vi "DopplerSVD_3D.vi"(0 "Choose Directory":path) -> ()   [LabVIEW 2022 SP3]
uses:
  <vilib>/Analysis/NI_AALPro.lvlib
  <vilib>/Analysis/Matrix/NI_Matrix.lvlib
  <vilib>/Analysis/Matrix/Numeric/Conversions/Matrix To Array - CM.vi
  <vilib>/Analysis/2dsp.llb/Complex FFT.vi
panel:
  in  "ms between frames":u32=100
  in  "Calc Spec Peaks":bool
  in  "animate":bool
  out "Peak V":sgl[][](graph)
  in  "read?":bool
  out "Waveform Graph":dbl[](graph)
  out "Complex output array":csg[][][](array[numeric])
  in  "image to display":i32
  in  "SV cut off":i32
  in  "stop":bool
  out "Raw data":dbl[][](graph)
  in  "Window Increment":i32=64
  in  "Window length":i32=64
  out "Doppler Signal":dbl[][](graph)
  in  "Parse":u16=1
  in  "Filter Prams":T1={"low cutoff"=5, "order"=81, "high cutoff"=35}
  in  "Type of Mean":u16(ring)=3 items=["Mean from lines", "Mean just lines", "Poly Mean", "No mean", "Filter"]
  in  "file ext":string="*IQSum_B3*"
  out "Numeric":i32
  in  "Use Selected Files":bool
  in  "Listbox":i32[](listbox)
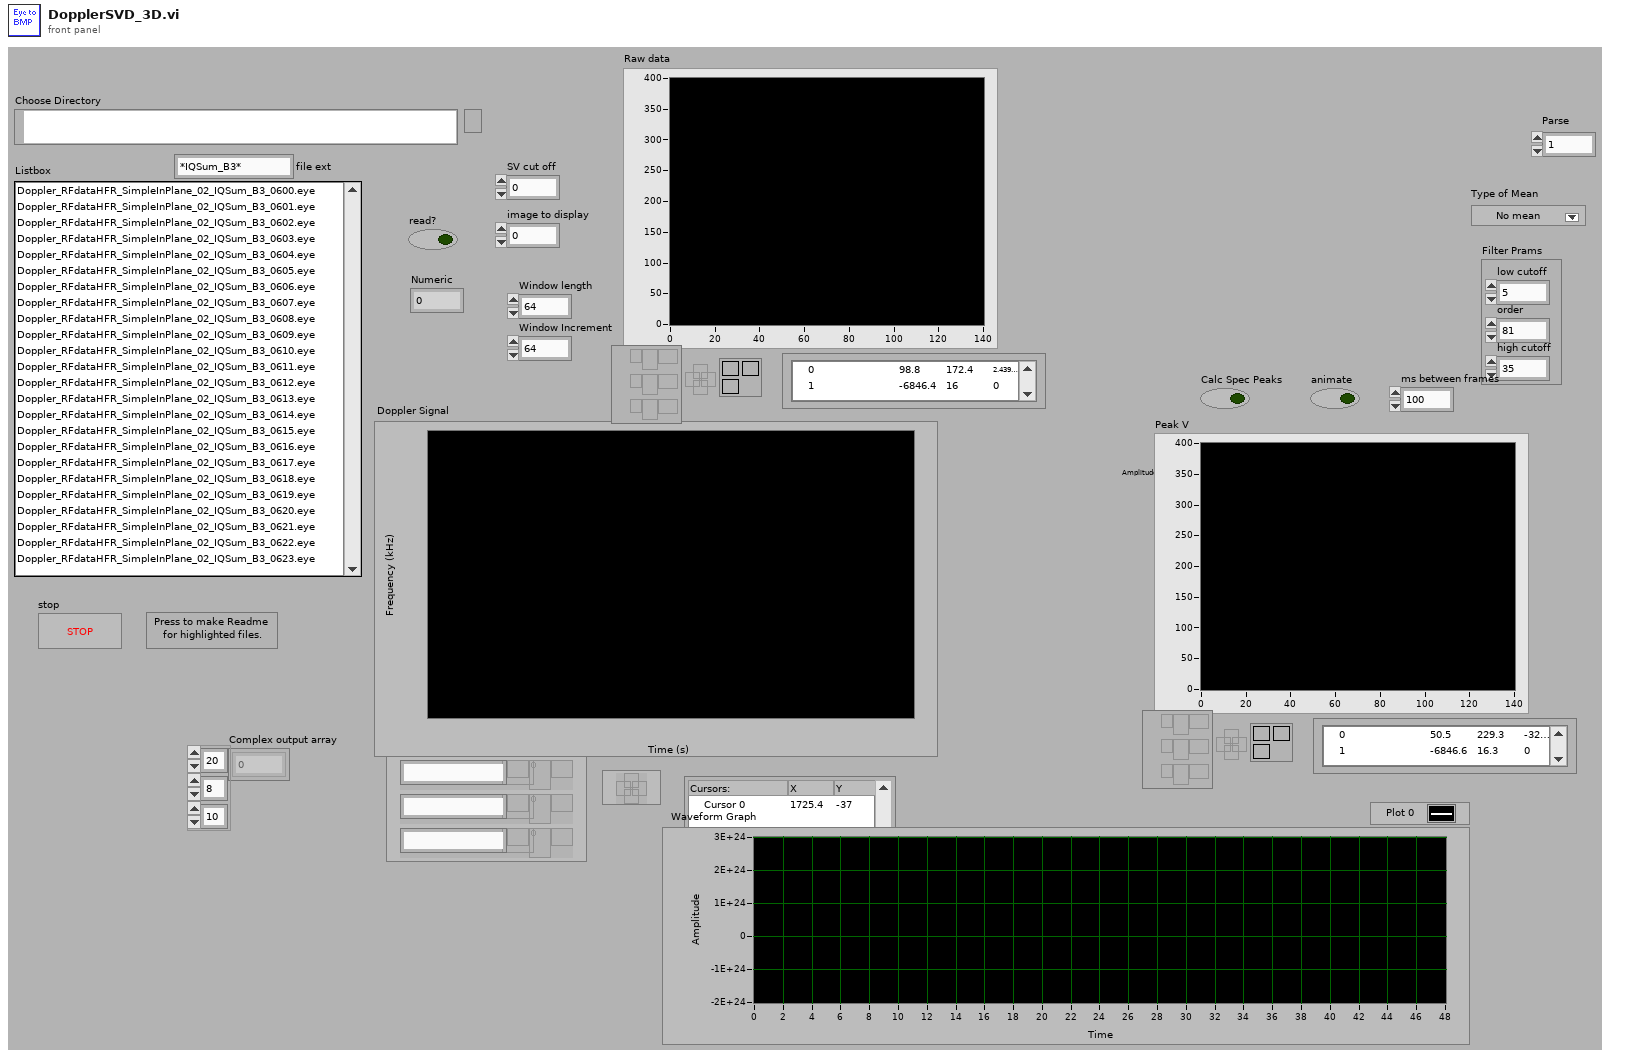
[diagram p1: front panel]
types:
  T1 = cluster{"low cutoff":i32, "order":i32, "high cutoff":i32}
  T2 = typedef "Header.ctl" = cluster{"header info":cluster{"Header":string, "Head length":i16}, "A/D info":cluster{"# rf points per line":u16, "# lines per scan":u16, "sample rate MHz":u16, "# A/D bits":i16, "# bytes per A/D":u16, "TGC Flag":u16, "A/D Type":string}, "Tranducer Info":cluster{"bandwidth":sgl, "center freq":sgl, "start freq":sgl, "ID":i32}, "Scan Info":cluster{"delay":sgl, "pivot distance":sgl, "sector scan angle":sgl, "operator":string, "Scan Mode":string, "location":string}, "Time/Date Info":cluster{"date":string, "time":string}, "RF Info":cluster{"RF file name":string, "RF file att":string, "RF cal file name":string, "RF cal file att":string}, "Patient Info":cluster{"ID":string, "extended ID":string, "age":u16, "sex":string, "previously\nscanned":string, "PSA":sgl, "LOS":u8, "Ethnicty 2":u8, "Race":u8}, "Tissue Type":cluster{"organ":i16, "disease type":i16, "disease location":i16, "IQ_pts":u16, "RcvBuffer":u8, "RcvFrame":u16, "IQBuff":u8, "IQFrame":u16, "IQPage":u8}, "Votage scaling":cluster{"Digitizer (dB)":sgl, "Gain (dB)":sgl, "Atten (dB)":sgl}, "Comment":string, "Misc Info":cluster{"avg num":u16, "c speed":i16, "Div By or SF zones":i16, "XMIT CHS":u8, "RCV CHS":u8, "Xmit angle":sgl}, "Therapy Parameters":cluster{"Theraputic Freq (MHz)":sgl, "Time on (s)":sgl, "Therapy amplitude (mV)":sgl, "Lines Before":u16, "Lines After":u16}, "Scan Settings":cluster{"Energy (uJ or V)":u8, "Damp (Ohm) or Fc":u8, "HP Filt (KHz)":u8, "LP Filt (MHz)":u8, "Gain (db)":u8, "prf (kHz)":sgl, "Distance between\nscan lines (um)":u16, "Distance between\nscan planes (um)":u16, "Scan line gap (um)":sgl, "Scan plane gap (um)":sgl}, "Compression Parameters":cluster{"F1 (MHz)":sgl, "F2 (MHz)":sgl, "% taper":sgl, "duration":sgl}, "Patient Info Xtra":cluster{"First Name":string, "Last Name":string, "Notes":string}, "ROI Box":u16[]}
  T3 = cluster{cluster{dbl, u16}, dbl, dbl, "delay":sgl, "delay":sgl, dbl, dbl}
  T4 = typedef "NI_Matrix.lvlib/ComplexMatrix.ctl" = cdb[][]
  T5 = cluster{"Vector S":cdb[], "Matrix V":T4, "Spectra":dbl[][], "indexes":i32[]}
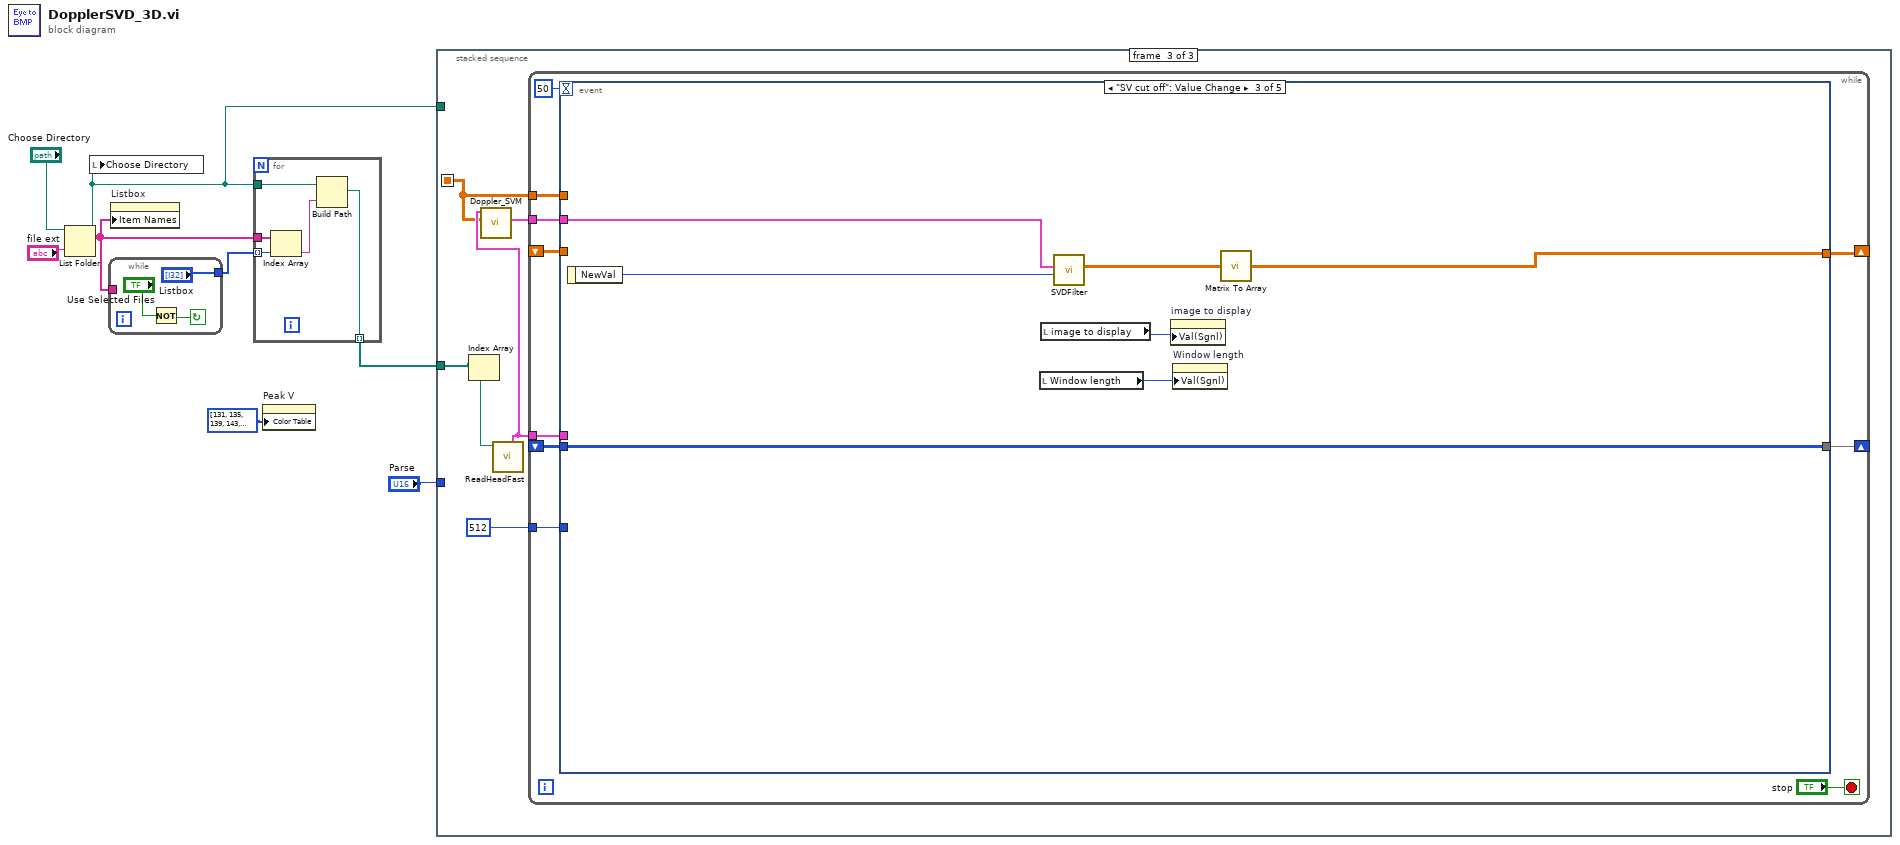
[diagram p0: block diagram]
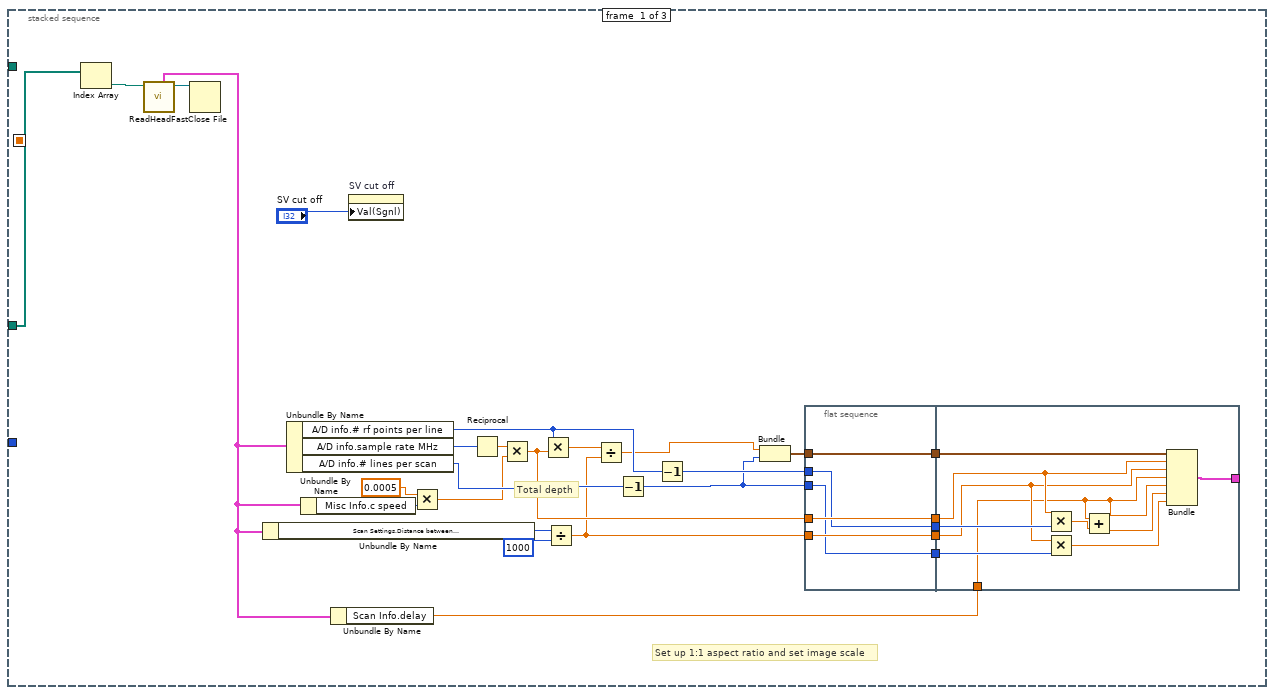
[diagram p2: hidden frame]
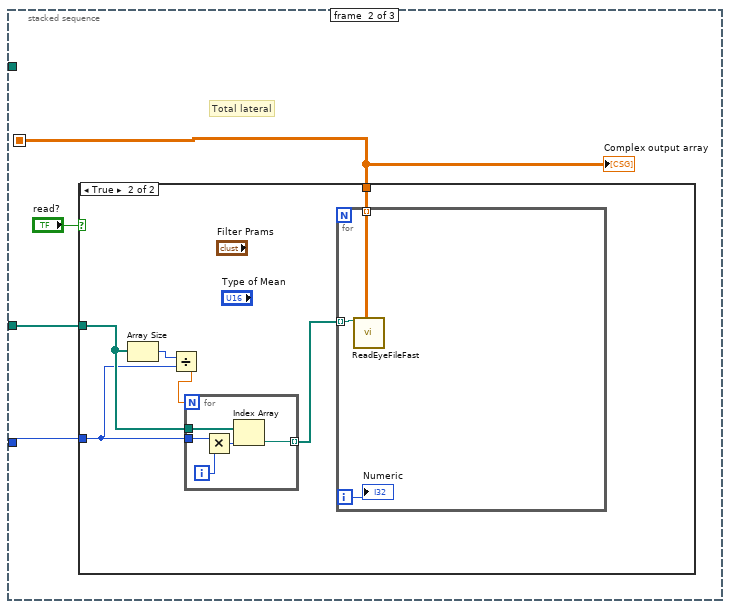
[diagram p3: hidden frame]
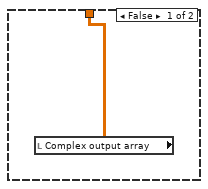
[diagram p4: hidden frame]
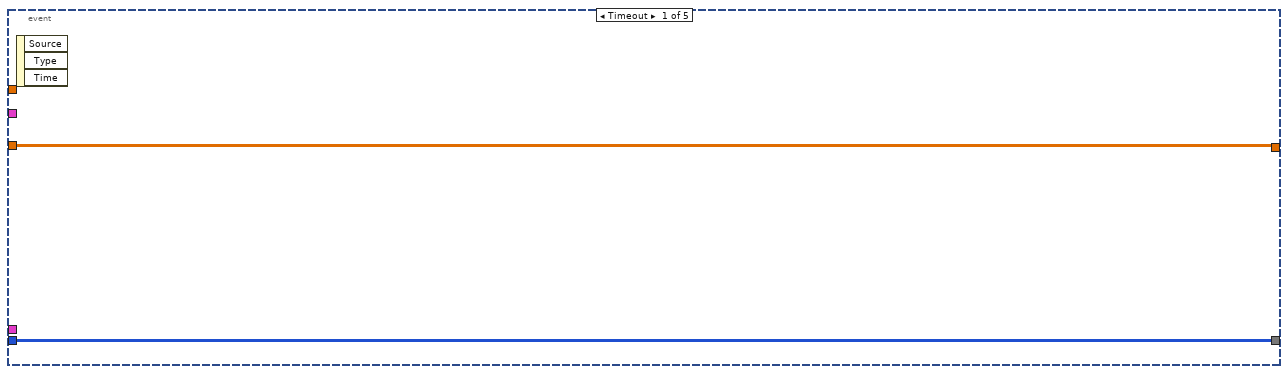
[diagram p5: hidden frame]
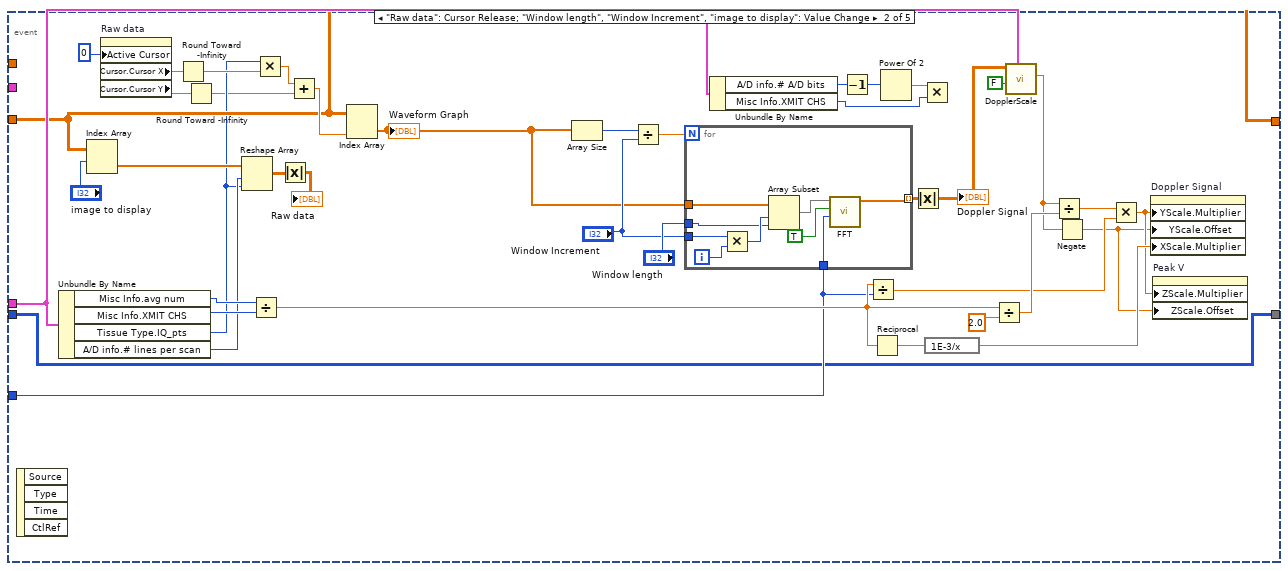
[diagram p6: hidden frame]
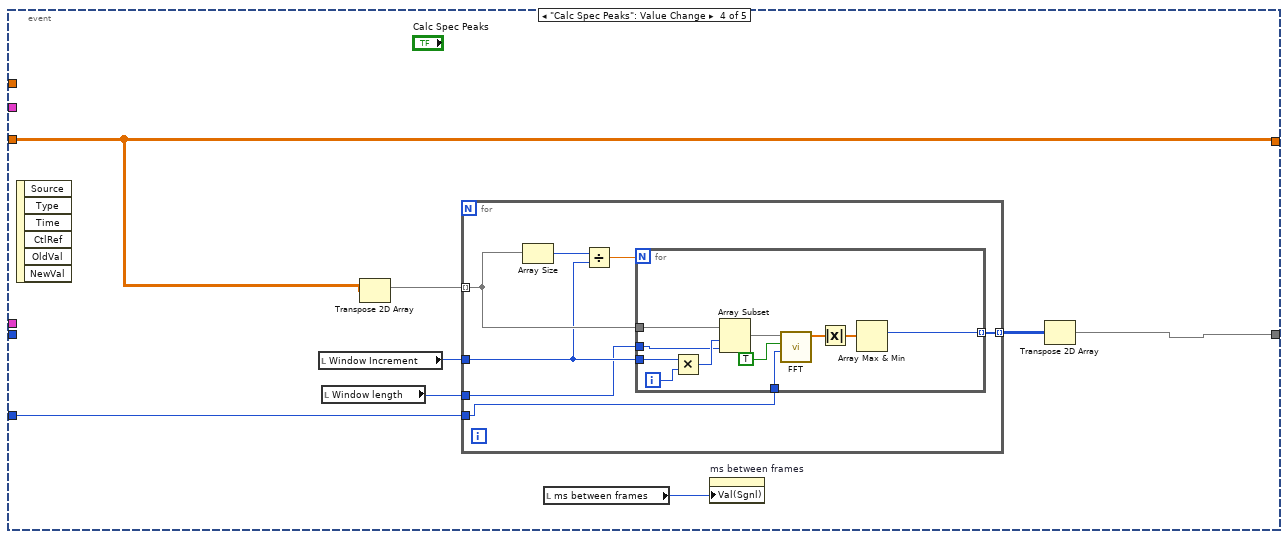
[diagram p7: hidden frame]
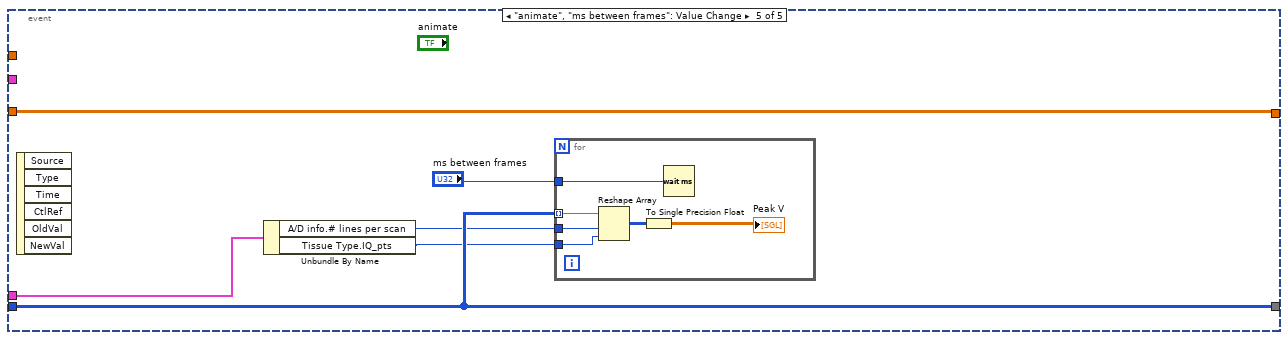
[diagram p8: hidden frame]
diagram:
  n1 = List Folder(path="Choose Directory", pattern="file ext") -> (path out=w5:path, filenames=w8:string[])  [unwired: 1 in, 3 out]
  n2 = local write "Choose Directory"(w5) -> ()
  n3 = while {
    tunnel: ["Listbox"] -> w7
    tunnel: w8 -> [_]
    stop <- w11 continue-if-true
    n4 = Not(x="Use Selected Files") -> (.not. x?=w11:bool)
  }
  n5 = property on="Listbox" class="LstBox (strict)"("Item Names"=w8) -> ()  [unwired: 2 in, 2 out]
  n6 = for {
    tunnel: w8 -> [w16]
    tunnel: w7 -> [w15] mode=indexing
    tunnel: [w12] -> w2 mode=indexing
    tunnel: w5 -> [w13]
    n7 = Index Array(array=w16, index=w15) -> (element=w14:string)
    n8 = Build Path(base path=w13, name or relative path=w14) -> (appended path=w12:path)
  }
  n9 = property on="Peak V" class="IntGraph (strict)"("Color Table"=u32[] [131, 135, 139, 143, 147, 151, 155, 159, 163, 167, 171, 175, 179, 183, 187, 191, 195, 199, 203, 207, 211, 215, 219, 223, 227, 231, 235, 239, 243, 247, 251, 255, 1279, 2303, 3327, 4351, 5375, 6399, 7423, 8447, 9471, 10495, 11519, 12543, 13567, 14591, 15615, 16639, 17663, 18687, 19711, 20735, 21759, 22783, 23807, 24831, 25855, 26879, 27903, 28927, 29951, 30975, 31999, 33023, 33791, 34815, 35839, 36863, 37887, 38911, 39935, 40959, 41983, 43007, 44031, 45055, 46079, 47103, 48127, 49151, 50175, 51199, 52223, 53247, 54271, 55295, 56319, 57343, 58367, 59391, 60415, 61439, 62463, 63487, 64511, 65535, 327675, 589815, 851955, 1114095, 1376235, 1638375, 1900515, 2162655, 2424795, 2686935, 2949075, 3211215, 3473355, 3735495, 3997635, 4259775, 4521915, 4784055, 5046195, 5308335, 5570475, 5832615, 6094755, 6356895, 6619035, 6881175, 7143315, 7405455, 7667595, 7929735, 8191875, 8454016, 8650620, 8912760, 9174900, 9437040, 9699180, 9961320, 10223460, 10485600, 10747740, 11009880, 11272020, 11534160, 11796300, 12058440, 12320580, 12582720, 12844860, 13107000, 13369140, 13631280, 13893420, 14155560, 14417700, 14679840, 14941980, 15204120, 15466260, 15728400, 15990540, 16252680, 16514820, 16776960, 16775936, 16774912, 16773888, 16772864, 16771840, 16770816, 16769792, 16768768, 16767744, 16766720, 16765696, 16764672, 16763648, 16762624, 16761600, 16760576, 16759552, 16758528, 16757504, 16756480, 16755456, 16754432, 16753408, 16752384, 16751360, 16750336, 16749312, 16748288, 16747264, 16746240, 16745216, 16744448, 16743424, 16742400, 16741376, 16740352, 16739328, 16738304, 16737280, 16736256, 16735232, 16734208, 16733184, 16732160, 16731136, 16730112, 16729088, 16728064, 16727040, 16726016, 16724992, 16723968, 16722944, 16721920, 16720896, 16719872, 16718848, 16717824, 16716800, 16715776, 16714752, 16713728, 16712704, 16711680, 16449536, 16187392, 15925248, 15663104, 15400960, 15138816, 14876672, 14614528, 14352384, 14090240, 13828096, 13565952, 13303808, 13041664, 12779520, 12517376, 12255232, 11993088, 11730944, 11468800, 11206656, 10944512, 10682368, 10420224, 10158080, 9895936, 9633792, 9371648, 9109504, 8847360, 8585216, 8388608] ("Array")) -> ()  [unwired: 2 in, 2 out]
  n10 = stacked-sequence {
    seq-local: [_ w60 _] -> [_ _ w79]
    tunnel: w2 -> [w41 w62 w82]
    tunnel: w5 -> [_ _ _]
    tunnel: "Parse" -> [_ w61 _]
    frame #0 {
      # "Set up 1:1 aspect ratio and set image scale"
      # "Total depth"
      n11 = Index Array(array=w41) -> (element=w43:path)  [unwired: 1 in]
      n12 = call "ReadHeadFast.vi"("new file path"=w43) -> ("refnum out"=w42:refnum<file>, "Header In"=w40:T2)  [unwired: 7 in, 2 out]
      n13 = Close File(refnum=w42) -> ()  [unwired: 1 in, 2 out]
      n14 = Unbundle By Name(w40) -> ("Scan Settings.Distance between\nscan lines (um)"=w27:u16)
      n15 = Unbundle By Name(w40) -> ("A/D info.# rf points per line"=w30:u16, "A/D info.sample rate MHz"=w32:u16, "A/D info.# lines per scan"=w29:u16)
      n16 = Unbundle By Name(w40) -> ("Misc Info.c speed"=w26:i16)
      n17 = Unbundle By Name(w40) -> ("Scan Info.delay"=w22:sgl)
      n18 = property on="SV cut off" class="DigNum (strict)"("Val(Sgnl)"="SV cut off") -> ()  [unwired: 2 in, 2 out]
      n19 = Multiply(x=0.0005, y=w26) -> (x*y=w24:dbl)
      n20 = Reciprocal(x=w32) -> (1/x=w33:dbl)
      n21 = Multiply(x=w33, y=w24) -> (x*y=w23:dbl)
      n22 = Multiply(x=w30, y=w23) -> (x*y=w31:dbl)
      n23 = Divide(x=w27, y=1000) -> (x/y=w21:dbl)
      n24 = Divide(x=w31, y=w21) -> (x/y=w19:dbl)
      n25 = Decrement(x=w29) -> (x-1=w18:u16)
      n26 = Decrement(x=w30) -> (x-1=w28:u16)
      n27 = Bundle(w19, w18) -> (w20:cluster{dbl, u16})  [unwired: 1 out]
      n28 = flat-sequence {
        tunnel: w28 -> [w45]
        tunnel: w18 -> [w46]
        tunnel: w20 -> [w44]
        tunnel: [w48] -> w39
        tunnel: w23 -> [w48]
        tunnel: [w47] -> w38
        tunnel: w21 -> [w47]
        tunnel: [w46] -> w37
        tunnel: [w45] -> w36
        tunnel: [w44] -> w35
        tunnel: w39 -> [w54]
        tunnel: w22 -> [w52]
        tunnel: w38 -> [w53]
        tunnel: w37 -> [w58]
        tunnel: w36 -> [w57]
        tunnel: w35 -> [w55]
        tunnel: [w49] -> _
        frame #0 {
        }
        frame #1 {
          n29 = Multiply(x=w54, y=w57) -> (x*y=w56:dbl)
          n30 = Multiply(x=w53, y=w58) -> (x*y=w50:dbl)
          n31 = Add(x=w52, y=w56) -> (x+y=w51:dbl)
          n32 = Bundle(w55, w54, w53, "delay"=w52, "delay"=w52, w51, w50) -> (w49:T3)  [unwired: 1 out]
        }
      }
    }
    frame #1 {
      # "Total lateral"
      n33 = case shown="True" "read?" {
        tunnel: w62 -> [_ w67]
        tunnel: w61 -> [_ w64]
        tunnel: [w63 w65] -> w60
        frame False {
          n34 = local read "Complex output array"() -> (w63:csg[][][])
        }
        frame True {
          n35 = Array Size(array=w67) -> (size(s)=w69:i32)
          n36 = Divide(x=w69, y=w64) -> (x/y=w68:dbl)
          n37 = for {
            N: w68 -> [_]
            tunnel: w67 -> [w73]
            tunnel: w64 -> [w72]
            tunnel: [w71] -> w66 mode=indexing
            i -> [w74]
            n38 = Multiply(x=w72, y=w74) -> (x*y=w70:i32)
            n39 = Index Array(array=w73, index=w70) -> (element=w71:path)
          }
          n40 = for {
            tunnel: w66 -> [w77] mode=indexing
            tunnel: [w75] -> w65 mode=indexing
            i -> [w76]
            n41 = call "ReadEyeFileFast.vi"("new file path"=w77) -> ("Complex output array"=w75:csg[][])  [unwired: 1 in, 17 out]
            "Numeric" <- w76
          }
        }
      }
      "Complex output array" <- w60
    }
    frame #2 {
      n42 = Index Array(array=w82) -> (element=w83:path)  [unwired: 1 in]
      n43 = call "ReadHeadFast.vi"("new file path"=w83) -> ("Header In"=w81:T2)  [unwired: 7 in, 3 out]
      n44 = call "Doppler_SVM.vi"("Input Array"=w79, "Header In"=w81) -> ("output cluster"=w80:T5)  [unwired: 8 in, 1 out]
      n45 = while {
        tunnel: w81 -> [w91]
        tunnel: w80 -> [w90]
        shift-right: [w89] -> _
        shift-left: _ -> [w88]
        tunnel: w79 -> [w87]
        shift-right: [w86] -> _
        shift-left: _ -> [w85]
        tunnel: 512 ("FFT size") -> [w84]
        stop <- "stop" stop-if-true
        n46 = event shown="[2] \"SV cut off\": Value Change" {
          selector: _ -> [_ _ _ _ _]
          dyn-events: _ -> [_ _ _ _ _]
          timeout: 50 -> [_ _ _ _ _]
          tunnel: w91 -> [_ w114 _ _ w182]
          tunnel: w90 -> [_ _ w152 _ _]
          tunnel: [w95 w108 w147 w160 w184] -> w89
          tunnel: w88 -> [w95 w108 _ w160 w184]
          tunnel: w87 -> [_ _ _ _ _]
          tunnel: [w94 w96 w146 w154 w183] -> w86
          tunnel: w85 -> [w94 w96 w146 _ w183]
          tunnel: w84 -> [_ w97 _ w155 _]
          event Timeout {
            n47 = event-data() -> ()  [unwired: 1 in, 3 out]
          }
          event "Raw data": Cursor Release; "Window length", "Window Increment", "image to display": Value Change {
            n48 = event-data() -> ()  [unwired: 1 in, 4 out]
            n49 = Unbundle By Name(w114) -> ("Misc Info.avg num"=w118:u16, "Misc Info.XMIT CHS"=w128:u8, "Tissue Type.IQ_pts"=w103:u16, "A/D info.# lines per scan"=w106:u16)
            n50 = Index Array(array=w108, index (row)="image to display") -> (element=w113:cdb[])  [unwired: 1 in]
            n51 = property on="Raw data" class="IntGraph (strict)"("Active Cursor"=0 ("Cursor.Cursor Index")) -> ("Cursor.Cursor X"=w104:dbl, "Cursor.Cursor Y"=w102:dbl)  [unwired: 2 in, 2 out]
            n52 = Round Toward -Infinity(1:w104) -> (0:w105:dbl)
            n53 = Round Toward -Infinity(1:w102) -> (0:w101:dbl)
            n54 = Reshape Array(w113, w106, w103) -> (w107:cdb[][])
            n55 = Divide(x=w118, y=w128) -> (x/y=w115:dbl)
            n56 = Multiply(x=w103, y=w105) -> (x*y=w111:dbl)
            n57 = Absolute Value(x=w107) -> (abs(x)=→"Raw data":dbl[][])
            n58 = Add(x=w111, y=w101) -> (x+y=w110:dbl)
            n59 = Index Array(array=w108, index (col)=w110) -> (element=w100:cdb[])  [unwired: 1 in]
            "Waveform Graph" <- w100
            n60 = Array Size(array=w100) -> (size(s)=w132:i32)
            n61 = Divide(x=w132, y="Window Increment") -> (x/y=w130:dbl)
            n62 = for {
              N: w130 -> [_]
              tunnel: w100 -> [w145]
              tunnel: "Window length" -> [w140]
              tunnel: "Window Increment" -> [w143]
              tunnel: [w138] -> w117 mode=indexing
              tunnel: w97 -> [w139]
              i -> [w144]
              n63 = Multiply(x=w143, y=w144) -> (x*y=w142:i32)
              n64 = Array Subset(array=w145, index=w142, length=w140) -> (w137:cdb[])
              n65 = call-poly <vilib>:"FFT.vi"("FFT size"=w139, "shift?"=TRUE, "X"=w137) -> ("FFT {X}"=w138:cdb[])  [unwired: 7 in, 1 out]
            }
            n66 = Unbundle By Name(w114) -> ("A/D info.# A/D bits"=w127:i16, "Misc Info.XMIT CHS"=w124:u8)
            n67 = Decrement(x=w127) -> (x-1=w126:i16)
            n68 = Divide(x=w115, y=w97) -> (x/y=w121:dbl)
            n69 = Reciprocal(x=w115) -> (1/x=w136:dbl)
            n70 = Power Of 2(x=w126) -> (2^x=w125:dbl)
            n71 = Absolute Value(x=w117) -> (abs(x)=w116:dbl[][])
            "Doppler Signal" <- w116
            n72 = Multiply(x=w125, y=w124) -> ()  [unwired: 1 out]
            n73 = expression code="1E-3/x"(w136) -> (w129:dbl)
            n74 = Divide(x=w115, y=2.0) -> (x/y=w123:dbl)
            n75 = call "DopplerScale.vi"("Header In"=w114, "PRF1/2"=FALSE, "Velocity index in"=w116) -> ("max doppler velocity cm/s"=w120:dbl)  [unwired: 5 in, 3 out]
            n76 = Divide(x=w120, y=w123) -> (x/y=w122:dbl)
            n77 = Negate(x=w120) -> (-x=w98:dbl)
            n78 = Multiply(x=w122, y=w121) -> (x*y=w99:dbl)
            n79 = property on="Doppler Signal" class="IntGraph (strict)"("YScale.Multiplier"=w99, "YScale.Offset"=w98, "XScale.Multiplier"=w129) -> ()  [unwired: 2 in, 2 out]
            n80 = property on="Peak V" class="IntGraph (strict)"("ZScale.Multiplier"=w99, "ZScale.Offset"=w98) -> ()  [unwired: 2 in, 2 out]
          }
          event "SV cut off": Value Change {
            n81 = event-data() -> ("NewVal"=w151:i32)  [unwired: 1 in]
            n82 = local read "Window length"() -> (w150:i32)
            n83 = local read "image to display"() -> (w148:i32)
            n84 = call "SVDFilter.vi"("Low zero index"=w151, "output cluster"=w152) -> ("Filtered Output"=w149:cdb[][][])  [unwired: 8 in, 1 out]
            n85 = property on="image to display" class="DigNum (strict)"("Val(Sgnl)"=w148) -> ()  [unwired: 2 in, 2 out]
            n86 = property on="Window length" class="DigNum (strict)"("Val(Sgnl)"=w150) -> ()  [unwired: 2 in, 2 out]
            n87 = call-poly <vilib>:"Matrix To Array.vi"("Complex Matrix"=w149) -> ("Complex 2D Array"=w147:cdb[][])
          }
          event "Calc Spec Peaks": Value Change {
            n88 = event-data() -> ()  [unwired: 1 in, 6 out]
            n89 = local read "Window Increment"() -> (w158:i32)
            n90 = local read "Window length"() -> (w157:i32)
            n91 = Transpose 2D Array(2D array=w160) -> (transposed array=w159:cdb[][])
            n92 = for {
              tunnel: w159 -> [w166] mode=indexing
              tunnel: w158 -> [w165]
              tunnel: w157 -> [w164]
              tunnel: [w163] -> w156 mode=indexing
              tunnel: w155 -> [w161]
              n93 = Array Size(array=w166) -> (size(s)=w167:i32)
              n94 = Divide(x=w167, y=w165) -> (x/y=w162:dbl)
              n95 = for {
                N: w162 -> [_]
                tunnel: w166 -> [w178]
                tunnel: w164 -> [w173]
                tunnel: w165 -> [w176]
                tunnel: w161 -> [w172]
                tunnel: [w168] -> w163 mode=indexing
                i -> [w177]
                n96 = Multiply(x=w176, y=w177) -> (x*y=w175:i32)
                n97 = Array Subset(array=w178, index=w175, length=w173) -> (w171:cdb[])
                n98 = call-poly <vilib>:"FFT.vi"("FFT size"=w172, "shift?"=TRUE, "X"=w171) -> ("FFT {X}"=w170:cdb[])  [unwired: 7 in, 1 out]
                n99 = Absolute Value(x=w170) -> (abs(x)=w169:dbl[])
                n100 = Array Max & Min(array=w169) -> (max index (indices)=w168:i32)  [unwired: 3 out]
              }
            }
            n101 = local read "ms between frames"() -> (w153:u32)
            n102 = property on="ms between frames" class="DigNum (strict)"("Val(Sgnl)"=w153) -> ()  [unwired: 2 in, 2 out]
            n103 = Transpose 2D Array(2D array=w156) -> (transposed array=w154:i32[][])
          }
          event "animate", "ms between frames": Value Change {
            n104 = event-data() -> ()  [unwired: 1 in, 6 out]
            n105 = Unbundle By Name(w182) -> ("A/D info.# lines per scan"=w180:u16, "Tissue Type.IQ_pts"=w181:u16)
            n106 = for {
              tunnel: w183 -> [w190] mode=indexing
              tunnel: w180 -> [w189]
              tunnel: w181 -> [w188]
              tunnel: "ms between frames" -> [w185]
              n107 = Reshape Array(w190, w189, w188) -> (w187:i32[][])
              n108 = To Single Precision Float(number=w187) -> (single precision float=→"Peak V":sgl[][])
              n109 = Wait (ms)(milliseconds to wait=w185) -> ()  [unwired: 1 out]
            }
          }
        }
      }
    }
  }
